vi "Begin.vi"() -> (0 "error out":errorcluster)   [LabVIEW 2015]
doc: "Called before other user functions, this VI is expected to open initial I/O refnums, load in file data, and do all program initialization. Notice that the <B>error out</B> terminal is simply used for data flow. Wiring it to other structures or subVIs ensures that this VI runs first."
uses:
  Robot Global Data.vi
  <vilib>/Rock Robotics/WPI/DriverStation/WPI_DriverStationRobotMode2.ctl
  <vilib>/Rock Robotics/WPI/Counter/WPI_CounterDigitalInputToDigitalSource.vi
  <vilib>/Rock Robotics/SystemInterfaces/Typedef/FPGA_TypedefDigitalModule.ctl
  <vilib>/Rock Robotics/SystemInterfaces/DIO/FPGA_DIOChannel.ctl
  <vilib>/Rock Robotics/WPI/Encoder/WPI_EncoderType.ctl
  <vilib>/Rock Robotics/WPI/MotorControl/WPI_MotorControlOpen Talon.vi
  <vilib>/Rock Robotics/SystemInterfaces/DIO/FPGA_DIOPWMChannel.ctl
  <vilib>/Rock Robotics/WPI/SafetyOutput/WPI_SafetyOutputConfigMenu.ctl
  <vilib>/Rock Robotics/SystemInterfaces/AI/FPGA_AIGyroChannel.ctl
  <vilib>/Rock Robotics/WPI/RobotDrive/WPI_RobotDriveOpen2MotorWithTalon.vi
  <vilib>/Rock Robotics/WPI/Joystick/WPI_JoystickDeviceEnum.ctl
  <vilib>/Rock Robotics/SystemInterfaces/DIO/FPGA_DIORelayChannel.ctl
  <vilib>/Rock Robotics/WPI/Solenoid/WPI_SolenoidOpenDouble.vi
  <vilib>/Rock Robotics/SystemInterfaces/Typedef/FPGA_TypedefSolenoidModule.ctl
  <vilib>/Rock Robotics/WPI/Solenoid/WPI_SolenoidChannel.ctl
panel:
  out "error out 3":errorcluster
  out "error out 2":errorcluster
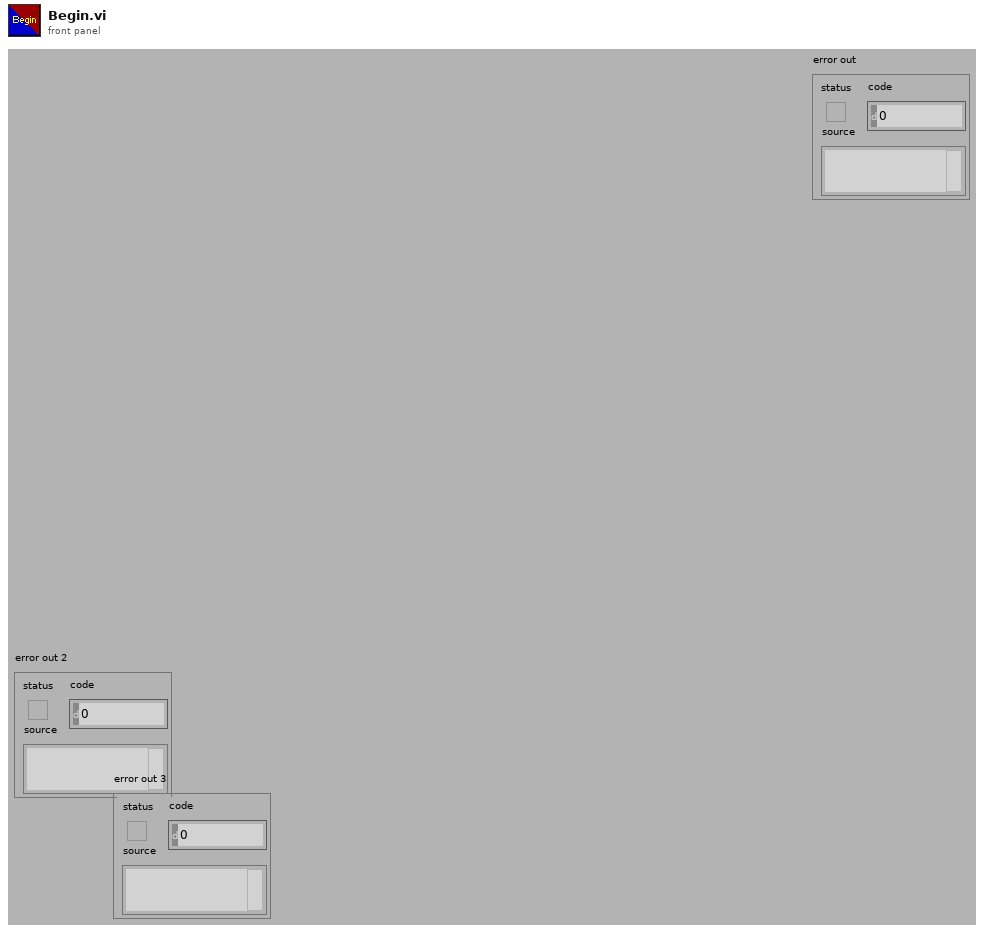
[diagram p1: front panel]
types:
  T1 = enum16{"Queen", "King", "Rook", "Knight", "Pawn"}
  T2 = typedef "WPI_SolenoidChannel.ctl" = enum8{"Solenoid 1", "Solenoid 2", "Solenoid 3", "Solenoid 4", "Solenoid 5", "Solenoid 6", "Solenoid 7", "Solenoid 8", "Invalid"}
  T3 = typedef "FPGA_TypedefSolenoidModule.ctl" = enum16{"Solenoid Module 1", "Solenoid Module 2"}
  T4 = typedef "FPGA_DIORelayChannel.ctl" = enum8{"Relay 1", "Relay 2", "Relay 3", "Relay 4", "Relay 5", "Relay 6", "Relay 7", "Relay 8", "Invalid"}
  T5 = typedef "FPGA_TypedefDigitalModule.ctl" = enum16{"Digital Module 1", "Digital Module 2"}
  T6 = typedef "FPGA_DIOChannel.ctl" = enum8{"DIO 1", "DIO 2", "DIO 3", "DIO 4", "DIO 5", "DIO 6", "DIO 7", "DIO 8", "DIO 9", "DIO 10", "DIO 11", "DIO 12", "DIO 13", "DIO 14", "Invalid"}
  T7 = typedef "FPGA_AIGyroChannel.ctl" = enum8{"AI 1", "AI 2", "Invalid"}
  T8 = typedef "WPI_SafetyOutputConfigMenu.ctl" = enum16{"Enable", "Disable"}
  T9 = typedef "FPGA_DIOPWMChannel.ctl" = enum8{"PWM 1", "PWM 2", "PWM 3", "PWM 4", "PWM 5", "PWM 6", "PWM 7", "PWM 8", "PWM 9", "PWM 10", "Invalid"}
  T10 = typedef "WPI_EncoderType.ctl" = enum16{"1x", "2x", "4x"}
  T11 = typedef "WPI_JoystickDeviceEnum.ctl" = enum16{"USB 0", "USB 1", "USB 2", "USB 3", "USB 4", "USB 5"}
  T12 = typedef "WPI_DriverStationRobotMode2.ctl" = enum16{"Autonomous Disabled", "Autonomous Enabled", "Teleop Disabled", "Teleop Enabled", "Disconnected", "Finish", "Test Disabled", "Test Enabled"}
  T13 = typedef "WPI_JoystickDevRef.ctl" = cluster{"Device":T11}
  T14 = typedef "WPI_RobotDriveDevRef.ctl" = cluster{"DevStatus":errorcluster, "Motors[]":T15[], "Square Inputs":bool, "Max Output":dbl}
  T15 = typedef "WPI_MotorControlDeviceRef.ctl" = cluster{"DeviceStatus":errorcluster, "Type":enum16{"PWM", "CAN"}, "PWM":cluster{"Digital Module":T5, "PWM Channel":T9, "DeadBand":T16}, "CAN":cluster{"Device Number":u8, "Control Mode":T17, "Semaphore":T18, "Max Vout":dbl}, "Invert":bool, "TransformRef":T19, "InvTransformRef":T19}
  T16 = typedef "WPI_PWMDeadband.ctl" = cluster{"Name":string, "maxPositivePwm":i32, "minPositivePwm":i32, "centerPwm":i32, "maxNegativePwm":i32, "minNegativePwm":i32, "angularRange":u16}
  T17 = typedef "WPI_CANJaguar_ControlMode.ctl" = enum8{"Percent VBus", "Current", "Speed", "Position", "Voltage"}
  T18 = typedef "Semaphore RefNum" = refnum<k1>
  T19 = typedef "WPI_PWMTransform_ConPane.ctl" = refnum<vi>
  T20 = typedef "WPI_DigitalInputDevRef.ctl" = cluster{"DevStatus":errorcluster, "DIO Channel":T6, "Digital Module":T5}
  T21 = typedef "FPGA_CounterEncoderSourceConvertionLVSourceType.ctl" = cluster{"DevStatus":errorcluster, "AnalogTriggerMode?":bool, "DigitalMode":cluster{"Digital Module":T5, "DIO Channel":T22}, "AnalogTriggerMode":cluster{"AnalogTriggerIndex":T23, "OutputType":T24}}
  T22 = typedef "FPGA_DIODigitalSourceChannel.ctl" = enum8{"DIO 1", "DIO 2", "DIO 3", "DIO 4", "DIO 5", "DIO 6", "DIO 7", "DIO 8", "DIO 9", "DIO 10", "DIO 11", "DIO 12", "DIO 13", "DIO 14", "Disabled"}
  T23 = typedef "FPGA_AnalogTriggerIndex.ctl" = enum8{"Trig 0", "Trig 1", "Trig 2", "Trig 3", "Trig 4", "Trig 5", "Trig 6", "Trig 7", "Invalid"}
  T24 = typedef "FPGA_AnalogTriggerOutType.ctl" = enum16{"InWindow", "TriggerState", "Rising", "Falling"}
  T25 = typedef "WPI_EncoderDevRef.ctl" = cluster{"DevStatus":errorcluster, "EncoderIndex":T26, "CounterIndex":T27, "DistancePerCount":dbl, "Decoding Type":T10}
  T26 = typedef "FPGA_EncoderIdx.ctl" = enum8{"Enc 0", "Enc 1", "Enc 2", "Enc 3", "Invalid"}
  T27 = typedef "FPGA_CounterCtrSystemIndex.ctl" = enum8{"Ctr 0", "Ctr 1", "Ctr 2", "Ctr 3", "Ctr 4", "Ctr 5", "Ctr 6", "Ctr 7", "Invalid"}
  T28 = typedef "WPI_GyroDevRef.ctl" = cluster{"DevStatus":errorcluster, "Analog Module":T29, "Analog Channel":T30, "Offset":dbl, "Gain (VoltsPerDegree/Second)":dbl}
  T29 = typedef "FPGA_TypedefAnalogModule.ctl" = enum16{"Analog Module 1", "Analog Module 2"}
  T30 = typedef "FPGA_AIChannel.ctl" = enum8{"AI 1", "AI 2", "AI 3", "AI 4", "AI 5", "AI 6", "AI 7", "AI 8", "Invalid"}
  T31 = typedef "WPI_CompressorDevRef.ctl" = cluster{"DevStatus":errorcluster, "DigitalInputDevRef":T20, "RelayDevRef":T32}
  T32 = typedef "WPI_RelayDevRef.ctl" = cluster{"DevStatus":errorcluster, "Relay Channel":T4, "Digital Module":T5, "Relay Direction":T33}
  T33 = typedef "WPI_RelayDirection.ctl" = enum16{"Both directions", "Forward only", "Reverse only"}
  T34 = typedef "WPI_SolenoidDevRef.ctl" = cluster{"DevStatus":errorcluster, "Solenoid Module":T3, "Forward Solenoid Channel":T2, "Reverse Solenoid Channel":T2}
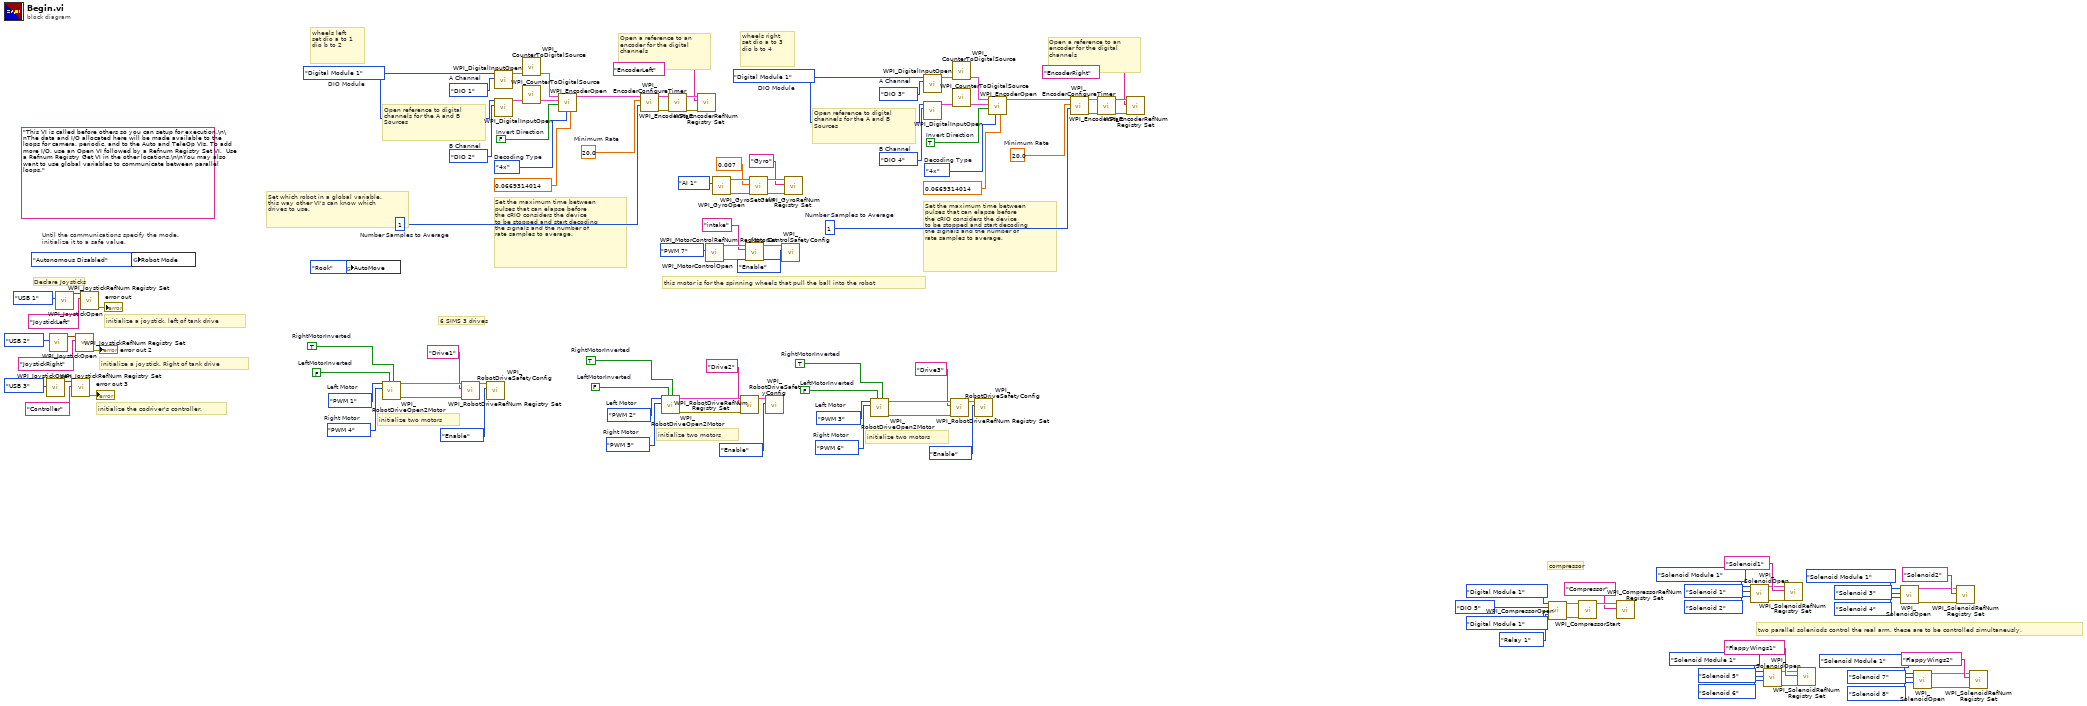
[diagram p0: block diagram]
diagram:
  w49 = FPGA_DIOPWMChannel."PWM 6"  # Right Motor
  w50 = FPGA_DIOPWMChannel."PWM 3"  # Left Motor
  w54 = FALSE  # LeftMotorInverted
  w55 = TRUE  # RightMotorInverted
  w58 = FPGA_DIOPWMChannel."PWM 5"  # Right Motor
  w59 = FPGA_DIOPWMChannel."PWM 2"  # Left Motor
  w63 = FALSE  # LeftMotorInverted
  w64 = TRUE  # RightMotorInverted
  w71 = u8 1  # Number Samples to Average
  w72 = 20.0  # Minimum Rate
  w76 = WPI_EncoderType."4x"  # Decoding Type
  w75 = TRUE  # Invert Direction
  w77 = FPGA_DIOChannel."DIO 4"  # B Channel
  w78 = FPGA_DIOChannel."DIO 3"  # A Channel
  w70 = FPGA_TypedefDigitalModule."Digital Module 1"  # DIO Module
  w89 = u8 1  # Number Samples to Average
  w90 = 20.0  # Minimum Rate
  w94 = WPI_EncoderType."4x"  # Decoding Type
  w93 = FALSE  # Invert Direction
  w95 = FPGA_DIOChannel."DIO 2"  # B Channel
  w96 = FPGA_DIOChannel."DIO 1"  # A Channel
  w88 = FPGA_TypedefDigitalModule."Digital Module 1"  # DIO Module
  w103 = FPGA_DIOPWMChannel."PWM 4"  # Right Motor
  w104 = FPGA_DIOPWMChannel."PWM 1"  # Left Motor
  w108 = FALSE  # LeftMotorInverted
  w109 = TRUE  # RightMotorInverted
  (unwired) "This VI is called before others so you can setup for execution.\n\nThe data and I/O allocated here will be made available to the loops for camera, periodic, and to the Auto and TeleOp VIs. To add more I/O, use an Open VI followed by a Refnum Registry Set VI.  Use a Refnum Registry Get VI in the other locations.\n\nYou may also want to use global variables to communicate between parallel loops."
  # "two parallel soleniods control the real arm. these are to be controlled simultaneusly."
  # "compressor"
  # "Set which robot in a global variable.\nthis way other VI's can know which\ndrives to use."
  # "6 SIMS 3 drives"
  # "this motor is for the spinning wheels that pull the ball into the robot"
  # "initialize two motors"
  # "initialize two motors"
  # "wheels right\nset dio a to 3\ndio b to 4"
  # "Set the maximum time between\npulses that can elapse before \nthe cRIO considers the device \nto be stopped and start decoding\nthe signals and the number of\nrate samples to average."
  # "Open a reference to an\nencoder for the digital \nchannels"
  # "Open reference to digital \nchannels for the A and B\nSources"
  # "wheels left\nset dio a to 1\ndio b to 2"
  # "Set the maximum time between\npulses that can elapse before \nthe cRIO considers the device \nto be stopped and start decoding\nthe signals and the number of\nrate samples to average."
  # "Open a reference to an\nencoder for the digital \nchannels"
  # "Open reference to digital \nchannels for the A and B\nSources"
  # "initialize two motors"
  # "Declare Joysticks"
  # "initialize the codriver's controller."
  # "initialize a joystick. Right of tank drive"
  # "initialize a joystick. left of tank drive"
  # "Until the communications specify the mode,\ninitialize it to a safe value."
  n1 = call <vilib>:"WPI_JoystickOpen.vi"("JoystickDevice"=WPI_JoystickDeviceEnum."USB 3") -> ("JoystickDevRef"=w113:T13)  [unwired: 10 in]
  n2 = call <vilib>:"WPI_JoystickOpen.vi"("JoystickDevice"=WPI_JoystickDeviceEnum."USB 2") -> ("JoystickDevRef"=w117:T13)  [unwired: 10 in]
  n3 = call <vilib>:"WPI_JoystickOpen.vi"("JoystickDevice"=WPI_JoystickDeviceEnum."USB 1") -> ("JoystickDevRef"=w110:T13)  [unwired: 10 in]
  n4 = call <vilib>:"WPI_JoystickRefNum Registry Set.vi"("refnum name"="Controller", "JoystickDevRef"=w113) -> ("error out"=→"error out 3":errorcluster)  [unwired: 8 in, 1 out]
  n5 = call <vilib>:"WPI_JoystickRefNum Registry Set.vi"("refnum name"="JoystickRight", "JoystickDevRef"=w117) -> ("error out"=→"error out 2":errorcluster)  [unwired: 8 in, 1 out]
  n6 = call <vilib>:"WPI_JoystickRefNum Registry Set.vi"("refnum name"="JoystickLeft", "JoystickDevRef"=w110) -> ("error out"=→"error out":errorcluster)  [unwired: 8 in, 1 out]
  n7 = global write "Robot Global Data.vi" "Robot Mode"(WPI_DriverStationRobotMode2."Autonomous Disabled" ("Robot Mode")) -> ()
  n8 = global write "Robot Global Data.vi" "AutoMove"(T1."Rook" ("AutoMove")) -> ()
  n9 = call-poly <vilib>:"WPI_RobotDriveOpen2Motor.vi"("Right Motor Inverted"=w109, "Left Motor Inverted"=w108, "Right Motor"=w103, "Left Motor"=w104) -> ("error out"=w105:errorcluster, "RobotDriveDevRef"=w107:T14)  [unwired: 1 in, 5 out]
  n10 = call <vilib>:"WPI_RobotDriveRefNum Registry Set.vi"("error in (no error)"=w105, "refnum name"="Drive1", "RobotDriveDevRef"=w107) -> ("RobotDriveDevRef"=w102:T14)  [unwired: 8 out]
  n11 = call <vilib>:"WPI_RobotDriveSafetyConfig.vi"("mode"=WPI_SafetyOutputConfigMenu."Enable", "RobotDriveDevRef"=w102) -> ()  [unwired: 8 in, 2 out]
  n12 = call <vilib>:"WPI_DigitalInputOpen.vi"("DIO Channel"=w96, "Digital Module (Module 1)"=w88) -> ("DigitalInputDevRef"=w98:T20)  [unwired: 1 in, 8 out]
  n13 = call <vilib>:"WPI_DigitalInputOpen.vi"("DIO Channel"=w95, "Digital Module (Module 1)"=w88) -> ("DigitalInputDevRef"=w99:T20)  [unwired: 1 in, 8 out]
  n14 = call-poly <vilib>:"WPI_CounterToDigitalSource.vi"("DigitalInputDevRef"=w98) -> ("Digital Source"=w97:T21)  [unwired: 6 out]
  n15 = call-poly <vilib>:"WPI_CounterToDigitalSource.vi"("DigitalInputDevRef"=w99) -> ("Digital Source"=w100:T21)  [unwired: 6 out]
  n16 = call <vilib>:"WPI_EncoderOpen.vi"("DistancePerCount"=0.0669314014, "Decoding Type"=w94, "Invert Direction (False)"=w93, "BSource"=w100, "ASource"=w97) -> ("EncoderDevRef"=w91:T25)  [unwired: 3 in, 3 out]
  n17 = call <vilib>:"WPI_EncoderConfigureTimer.vi"("Number Samples to Average"=w89, "Minimum Rate"=w90, "EncoderDevRef"=w91) -> ("error out"=w86:errorcluster, "EncoderDevRef"=w92:T25)  [unwired: 1 in, 6 out]
  n18 = call-poly <vilib>:"WPI_RobotDriveOpen2Motor.vi"("Right Motor Inverted"=w64, "Left Motor Inverted"=w63, "Right Motor"=w58, "Left Motor"=w59) -> ("error out"=w60:errorcluster, "RobotDriveDevRef"=w62:T14)  [unwired: 1 in, 5 out]
  n19 = call <vilib>:"WPI_EncoderStart.vi"("error in (no error)"=w86, "EncoderDevRef"=w92) -> ("error out"=w85:errorcluster, "EncoderDevRef"=w87:T25)  [unwired: 8 out]
  n20 = call <vilib>:"WPI_EncoderRefNum Registry Set.vi"("error in (no error)"=w85, "refnum name"="EncoderLeft", "EncoderDevRef"=w87) -> ()  [unwired: 7 in, 2 out]
  n21 = call-poly <vilib>:"WPI_MotorControlOpen.vi"("PWM Channel"=FPGA_DIOPWMChannel."PWM 7") -> ("error out"=w44:errorcluster, "MotorControlDeviceRef"=w45:T15)  [unwired: 9 in]
  n22 = call <vilib>:"WPI_GyroOpen.vi"("Analog Channel"=FPGA_AIGyroChannel."AI 1") -> ("error out"=w38:errorcluster, "GyroDevRef"=w39:T28)  [unwired: 8 in, 1 out]
  n23 = call <vilib>:"WPI_RobotDriveRefNum Registry Set.vi"("error in (no error)"=w60, "refnum name"="Drive2", "RobotDriveDevRef"=w62) -> ("RobotDriveDevRef"=w57:T14)  [unwired: 8 out]
  n24 = call <vilib>:"WPI_MotorControlRefNum Registry Set.vi"("error in (no error)"=w44, "refnum name"="intake", "MotorControlDevRef"=w45) -> ("MotorControlDevRef"=w42:T15)  [unwired: 7 in, 1 out]
  n25 = call <vilib>:"WPI_GyroSetGain.vi"("error in (no error)"=w38, "Gain (VoltsPerDegree/Second)"=0.007, "GyroDevRef"=w39) -> ("error out"=w36:errorcluster, "GyroDevRef"=w35:T28)  [unwired: 7 in]
  n26 = call <vilib>:"WPI_RobotDriveSafetyConfig.vi"("mode"=WPI_SafetyOutputConfigMenu."Enable", "RobotDriveDevRef"=w57) -> ()  [unwired: 8 in, 2 out]
  n27 = call <vilib>:"WPI_MotorControlSafetyConfig.vi"("mode"=WPI_SafetyOutputConfigMenu."Enable", "MotorControlDevRef"=w42) -> ()  [unwired: 8 in, 2 out]
  n28 = call <vilib>:"WPI_GyroRefNum Registry Set.vi"("error in (no error)"=w36, "refnum name"="Gyro", "GyroDevRef"=w35) -> ()  [unwired: 7 in, 2 out]
  n29 = call-poly <vilib>:"WPI_RobotDriveOpen2Motor.vi"("Right Motor Inverted"=w55, "Left Motor Inverted"=w54, "Right Motor"=w49, "Left Motor"=w50) -> ("error out"=w51:errorcluster, "RobotDriveDevRef"=w53:T14)  [unwired: 1 in, 5 out]
  n30 = call <vilib>:"WPI_DigitalInputOpen.vi"("DIO Channel"=w78, "Digital Module (Module 1)"=w70) -> ("DigitalInputDevRef"=w80:T20)  [unwired: 1 in, 8 out]
  n31 = call <vilib>:"WPI_DigitalInputOpen.vi"("DIO Channel"=w77, "Digital Module (Module 1)"=w70) -> ("DigitalInputDevRef"=w81:T20)  [unwired: 1 in, 8 out]
  n32 = call <vilib>:"WPI_RobotDriveRefNum Registry Set.vi"("error in (no error)"=w51, "refnum name"="Drive3", "RobotDriveDevRef"=w53) -> ("RobotDriveDevRef"=w48:T14)  [unwired: 8 out]
  n33 = call-poly <vilib>:"WPI_CounterToDigitalSource.vi"("DigitalInputDevRef"=w80) -> ("Digital Source"=w79:T21)  [unwired: 6 out]
  n34 = call-poly <vilib>:"WPI_CounterToDigitalSource.vi"("DigitalInputDevRef"=w81) -> ("Digital Source"=w82:T21)  [unwired: 6 out]
  n35 = call <vilib>:"WPI_RobotDriveSafetyConfig.vi"("mode"=WPI_SafetyOutputConfigMenu."Enable", "RobotDriveDevRef"=w48) -> ()  [unwired: 8 in, 2 out]
  n36 = call <vilib>:"WPI_EncoderOpen.vi"("DistancePerCount"=0.0669314014, "Decoding Type"=w76, "Invert Direction (False)"=w75, "BSource"=w82, "ASource"=w79) -> ("EncoderDevRef"=w73:T25)  [unwired: 3 in, 3 out]
  n37 = call <vilib>:"WPI_EncoderConfigureTimer.vi"("Number Samples to Average"=w71, "Minimum Rate"=w72, "EncoderDevRef"=w73) -> ("error out"=w68:errorcluster, "EncoderDevRef"=w74:T25)  [unwired: 1 in, 6 out]
  n38 = call <vilib>:"WPI_EncoderStart.vi"("error in (no error)"=w68, "EncoderDevRef"=w74) -> ("error out"=w67:errorcluster, "EncoderDevRef"=w69:T25)  [unwired: 8 out]
  n39 = call <vilib>:"WPI_EncoderRefNum Registry Set.vi"("error in (no error)"=w67, "refnum name"="EncoderRight", "EncoderDevRef"=w69) -> ()  [unwired: 7 in, 2 out]
  n40 = call <vilib>:"WPI_CompressorOpen.vi"("Pressure Switch Digital Module (Module 1)"=FPGA_TypedefDigitalModule."Digital Module 1", "Pressure Switch DIO Channel"=FPGA_DIOChannel."DIO 5", "Relay Digital Module (Module 1)"=FPGA_TypedefDigitalModule."Digital Module 1", "Relay Channel"=FPGA_DIORelayChannel."Relay 1") -> ("CompressorDevRef"=w33:T31, "error out"=w31:errorcluster)  [unwired: 10 in]
  n41 = call <vilib>:"WPI_CompressorStart.vi"("error in (no error)"=w31, "CompressorDevRef"=w33) -> ("CompressorDevRef"=w32:T31)  [unwired: 8 in, 1 out]
  n42 = call <vilib>:"WPI_CompressorRefNum Registry Set.vi"("refnum name"="Compressor", "CompressorDevRef"=w32) -> ()  [unwired: 8 in, 2 out]
  n43 = call-poly <vilib>:"WPI_SolenoidOpen.vi"("Reverse Solenoid Channel"=WPI_SolenoidChannel."Solenoid 2", "Forward Solenoid Channel"=WPI_SolenoidChannel."Solenoid 1", "Solenoid Module (Module 1)"=FPGA_TypedefSolenoidModule."Solenoid Module 1") -> ("error out"=w25:errorcluster, "SolenoidDevRef"=w26:T34)  [unwired: 7 in]
  n44 = call-poly <vilib>:"WPI_SolenoidOpen.vi"("Reverse Solenoid Channel"=WPI_SolenoidChannel."Solenoid 6", "Forward Solenoid Channel"=WPI_SolenoidChannel."Solenoid 5", "Solenoid Module (Module 1)"=FPGA_TypedefSolenoidModule."Solenoid Module 1") -> ("error out"=w8:errorcluster, "SolenoidDevRef"=w9:T34)  [unwired: 7 in]
  n45 = call <vilib>:"WPI_SolenoidRefNum Registry Set.vi"("error in (no error)"=w25, "refnum name"="Solenoid1", "SolenoidDevRef"=w26) -> ()  [unwired: 7 in, 2 out]
  n46 = call <vilib>:"WPI_SolenoidRefNum Registry Set.vi"("error in (no error)"=w8, "refnum name"="FlappyWings1", "SolenoidDevRef"=w9) -> ()  [unwired: 7 in, 2 out]
  n47 = call-poly <vilib>:"WPI_SolenoidOpen.vi"("Reverse Solenoid Channel"=WPI_SolenoidChannel."Solenoid 4", "Forward Solenoid Channel"=WPI_SolenoidChannel."Solenoid 3", "Solenoid Module (Module 1)"=FPGA_TypedefSolenoidModule."Solenoid Module 1") -> ("error out"=w29:errorcluster, "SolenoidDevRef"=w28:T34)  [unwired: 7 in]
  n48 = call-poly <vilib>:"WPI_SolenoidOpen.vi"("Reverse Solenoid Channel"=WPI_SolenoidChannel."Solenoid 8", "Forward Solenoid Channel"=WPI_SolenoidChannel."Solenoid 7", "Solenoid Module (Module 1)"=FPGA_TypedefSolenoidModule."Solenoid Module 1") -> ("error out"=w12:errorcluster, "SolenoidDevRef"=w11:T34)  [unwired: 7 in]
  n49 = call <vilib>:"WPI_SolenoidRefNum Registry Set.vi"("error in (no error)"=w29, "refnum name"="Solenoid2", "SolenoidDevRef"=w28) -> ()  [unwired: 7 in, 2 out]
  n50 = call <vilib>:"WPI_SolenoidRefNum Registry Set.vi"("error in (no error)"=w12, "refnum name"="FlappyWings2", "SolenoidDevRef"=w11) -> ()  [unwired: 7 in, 2 out]
